vi "Next State.vi"(10 "Manual":bool, 11 "Fault?":bool) -> (3 "String":string)   [LabVIEW 2014]
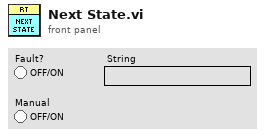
[diagram p1: front panel]
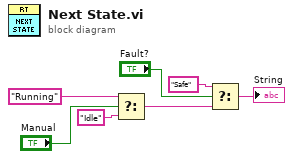
[diagram p0: block diagram]
diagram:
  n1 = Select(t="Running", s="Manual", f="Idle") -> (s? t:f=w3:string)
  n2 = Select(t="Safe", s="Fault?", f=w3) -> (s? t:f=→"String":string)
